vi "MultiStation@AddStation(Dynamic)__Parameter.vi"(1 "ParamterIn":string) -> (0 "ParamterOut":string)   [LabVIEW 2020]
panel:
  in  "Parameter":string(combo)
  in  "StationName":string(combo)
  in  "Confirm":bool
  # "MultiStation@General $Station(,ParameterS)"
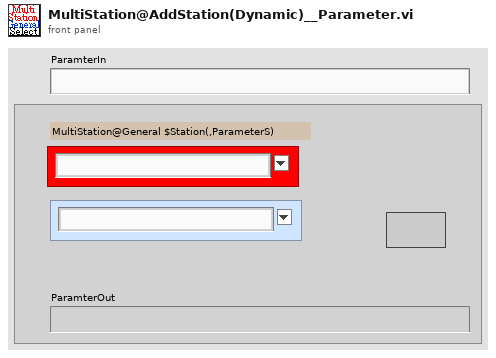
[diagram p1: front panel]
types:
  T1 = enum16{"Init", "AddStation", "StateShift", "ResetDefault", "SetStationON", "SetStationOFF", "SetStationOK", "SetStationNG", "UpdateIndicator", "SetData", "GetData", "GetOnOff", "GetOkNg", "ShowFeedInTray", "ShowFeedOutTray", "BlinkingOn", "BlinkingOff"}
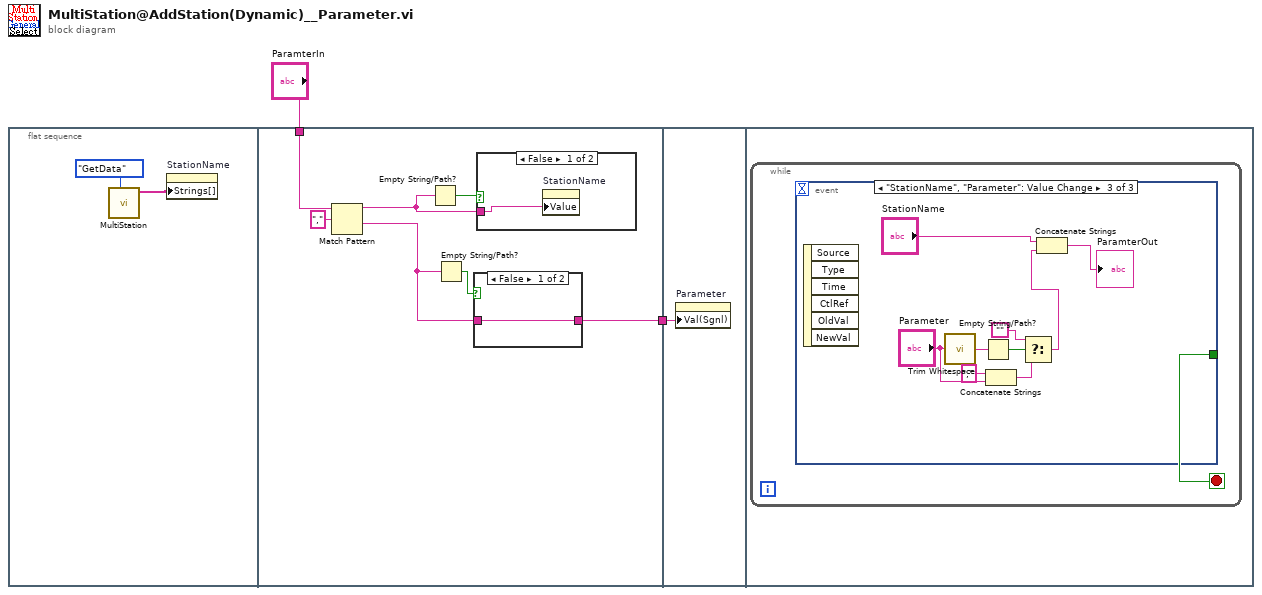
[diagram p0: block diagram]
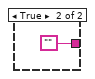
[diagram p2: hidden frame]
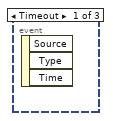
[diagram p4: hidden frame]
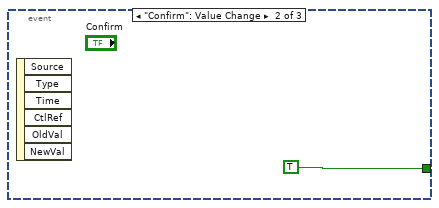
[diagram p5: hidden frame]
diagram:
  n1 = flat-sequence {
    tunnel: "ParamterIn" -> [w8]
    tunnel: [w9] -> w1
    tunnel: w1 -> [w15]
    frame #0 {
      n2 = call "MultiStation.vi"("OP"=T1."GetData") -> ("StationList"=w3:string[])  [unwired: 6 in, 4 out]
      n3 = property on="StationName" class="CmbBox"("Strings[]"=w3) -> ()  [unwired: 2 in, 2 out]
    }
    frame #1 {
      n4 = Match Pattern(string=w8, regular expression="," ("search string")) -> (before substring=w5:string, after substring=w6:string)  [unwired: 1 in, 2 out]
      n5 = Empty String/Path?(string/path=w5) -> (empty?=w11:bool)
      n6 = Empty String/Path?(string/path=w6) -> (empty?=w10:bool)
      n7 = case shown="False" w10 {
        tunnel: [w12 ""] -> w9
        tunnel: w6 -> [w12 _]
        frame False {
        }
        frame True {
        }
      }
      n8 = case shown="False" w11 {
        tunnel: w5 -> [w14 _]
        frame False {
          n9 = property on="StationName" class="CmbBox"("Value"=w14) -> ()  [unwired: 2 in, 2 out]
        }
        frame True {
        }
      }
    }
    frame #2 {
      n10 = property on="Parameter" class="CmbBox"("Val(Sgnl)"=w15) -> ()  [unwired: 2 in, 2 out]
    }
    frame #3 {
      n11 = while {
        stop <- w16 stop-if-true
        n12 = event shown="[2] \"StationName\", \"Parameter\": Value Change" {
          selector: _ -> [_ _ _]
          dyn-events: _ -> [_ _ _]
          timeout: _ -> [_ _ _]
          tunnel: [_ TRUE _] -> w16
          event Timeout {
            n13 = event-data() -> ()  [unwired: 1 in, 3 out]
          }
          event "Confirm": Value Change {
            n14 = event-data() -> ()  [unwired: 1 in, 6 out]
          }
          event "StationName", "Parameter": Value Change {
            n15 = event-data() -> ()  [unwired: 1 in, 6 out]
            n16 = call <vilib>:"Trim Whitespace.vi"("string"="Parameter") -> ("trimmed string"=w21:string)  [unwired: 1 in]
            n17 = Empty String/Path?(string/path=w21) -> (empty?=w22:bool)
            n18 = Concatenate Strings("," ("string"), "Parameter") -> (w24:string)
            n19 = Select(t="", s=w22, f=w24) -> (s? t:f=w19:string)
            n20 = Concatenate Strings("StationName", w19) -> (→"ParamterOut":string)
          }
        }
      }
    }
  }
